vi "IsSinglePoint.vi"(11 "MeasType":string) -> (2 "is single point":bool)   [LabVIEW 2017, in "DeviceModelHelpers.lvlib"]
uses:
  <vilib>/addons/InsightCM/Utilities/DeviceModelHelpers/DeviceModelHelpers.lvlib
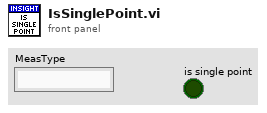
[diagram p1: front panel]
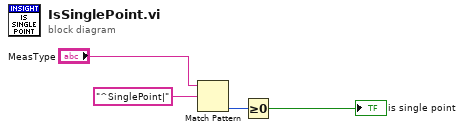
[diagram p0: block diagram]
diagram:
  n1 = Match Pattern(string="MeasType", regular expression="^SinglePoint|") -> (offset past match=w1:i32)  [unwired: 1 in, 3 out]
  n2 = Greater Or Equal To 0?(x=w1) -> (x >= 0?=→"is single point":bool)
